vi "Write Transmission Data Unit.vi"(8 "error in (no error)":errorcluster, 10 "Transmission Data Unit":refnum<class "Transmission Data Unit.lvclass">, 11 "Network Master in":refnum<class "Network Master.lvclass">) -> (0 "error out":errorcluster, 3 "Network Master out":refnum<class "Network Master.lvclass">)   [LabVIEW 2021, in "Network Master.lvclass"]
uses:
  Network Master.lvclass
  Transmission Data Unit/Transmission Data Unit.lvclass
  Network Master.lvclass/Network Master.ctl
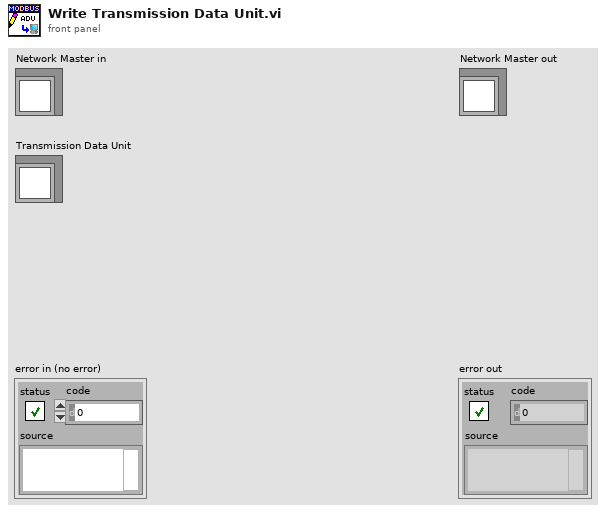
[diagram p1: front panel]
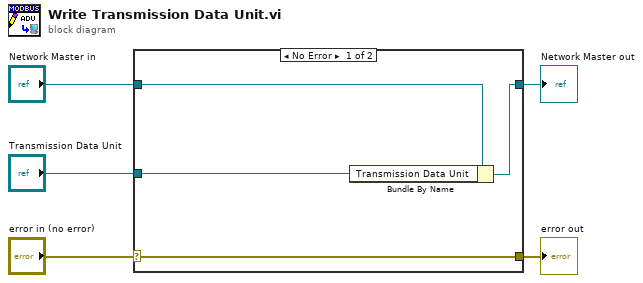
[diagram p0: block diagram]
diagram:
  n1 = case shown="No Error" "error in (no error)" {
    selector: "error in (no error)" -> [w9 w10]
    tunnel: [w9 w10] -> w4
    tunnel: [w7 w11] -> w2
    tunnel: "Network Master in" -> [w8 w11]
    tunnel: "Transmission Data Unit" -> [w6 _]
    frame No Error {
      n2 = Bundle By Name(cluster=w8, "Transmission Data Unit"=w6) -> (w7:refnum<class "Network Master.lvclass">)
    }
    frame Error {
    }
  }
  "error out" <- w4
  "Network Master out" <- w2
